vi "StartTestSuite_AfterStartTestSuite_AddsNestedTestSuite.vi"() -> (0 "error out":errorcluster)   [LabVIEW 2017, in "ResultTreeListenerTest.lvlib"]
uses:
  ResultTreeListenerTest.lvlib
  ResultTreeListener/ResultTreeListener.lvclass
  ResultTree/ResultTree.lvclass
  Support/FakeTestSuite/FakeTestSuite.lvclass
  6b75ad31-72ea-41ab-b928-28c96779d91c.vi
  C:/Users/de200256/Code/neuperger/lvunit/TestSuite/TestSuite.lvclass
panel:
  in  "Tree":string(tree)
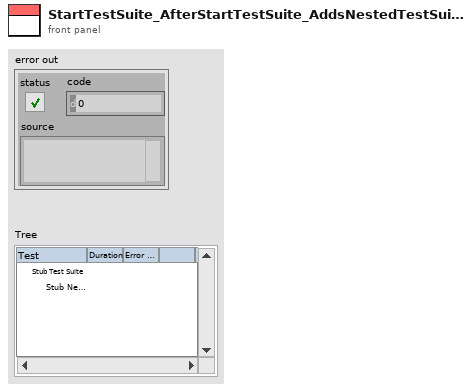
[diagram p1: front panel]
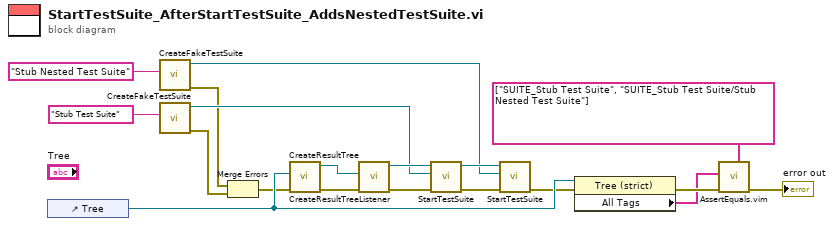
[diagram p0: block diagram]
diagram:
  n1 = control-ref of="Tree"() -> (w11:refnum<vi>)
  n2 = call "CreateFakeTestSuite.vi"("Name"="Stub Nested Test Suite") -> ("error out"=w2:errorcluster, "FakeTestSuite out"=w4:refnum<class "FakeTestSuite.lvclass">)  [unwired: 9 in]
  n3 = call "CreateFakeTestSuite.vi"("Name"="Stub Test Suite") -> ("error out"=w1:errorcluster, "FakeTestSuite out"=w14:refnum<class "FakeTestSuite.lvclass">)  [unwired: 9 in]
  n4 = Merge Errors(w2, w1) -> (w3:errorcluster)
  n5 = call "CreateResultTree.vi"("error in (no error)"=w3, "Tree Refnum"=w11) -> ("error out"=w19:errorcluster, "ResultTree out"=w18:refnum<class "ResultTree.lvclass">)  [unwired: 8 in]
  n6 = call "CreateResultTreeListener.vi"("error in (no error)"=w19, "ResultTree"=w18) -> ("error out"=w17:errorcluster, "ResultTreeListener out"=w15:refnum<class "ResultTreeListener.lvclass">)  [unwired: 8 in]
  n7 = call-dynamic "StartTestSuite.vi"("error in (no error)"=w17, "TestSuite"=w14, "ResultTreeListener in"=w15) -> ("error out"=w7:errorcluster, "ResultTreeListener out"=w5:refnum<class "ResultTreeListener.lvclass">)  [unwired: 7 in]
  n8 = call-dynamic "StartTestSuite.vi"("error in (no error)"=w7, "TestSuite"=w4, "ResultTreeListener in"=w5) -> ("error out"=w6:errorcluster)  [unwired: 7 in, 1 out]
  n9 = property class="Tree (strict)"(reference=w11, error in=w6) -> (error out=w12:errorcluster, "All Tags"=w10:string[])  [unwired: 1 out]
  n10 = call "AssertEquals.vim"("Expected"=string[] ["SUITE_Stub Test Suite", "SUITE_Stub Test Suite/Stub Nested Test Suite"] ("All Tags"), "error in (no error)"=w12, "Actual"=w10) -> ("error out"=→"error out":errorcluster)  [unwired: 8 in]
